vi "ReversedEngineering GetAdditionalTransitionStates.vi"(1 "SelStrings":string[](array[string]), 2 "StringConstant":string) -> (15 "AdditionalTransitionStates":string[](array[string]))   [LabVIEW 2020]
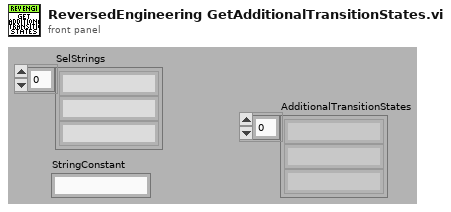
[diagram p1: front panel]
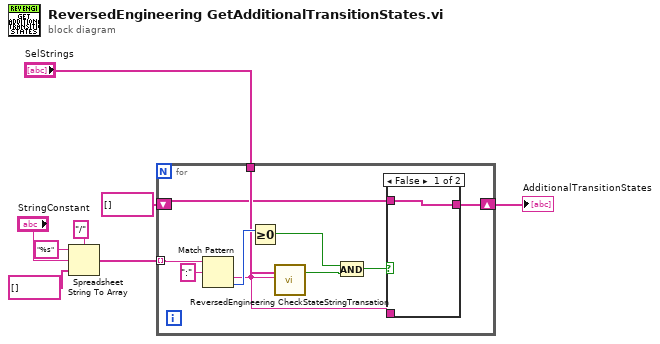
[diagram p0: block diagram]
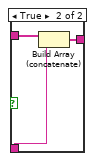
[diagram p2: hidden frame]
diagram:
  n1 = Spreadsheet String To Array(delimiter (Tab)="/", format string="%s", spreadsheet string="StringConstant", array type (2D Dbl)=string[] []) -> (array=w4:string[])
  n2 = for {
    tunnel: w4 -> [w17] mode=indexing
    tunnel: "SelStrings" -> [w15]
    shift-right: [w11] -> w1
    shift-left: string[] [] -> [w10]
    n3 = Match Pattern(string=w17, regular expression=":") -> (after substring=w9:string, offset past match=w16:i32)  [unwired: 3 out]
    n4 = Greater Or Equal To 0?(x=w16) -> (x >= 0?=w13:bool)
    n5 = call <resource>:"ReversedEngineering CheckStateStringTransation.vi"("SelStrings"=w15, "StringConstant"=w9) -> ("Found"=w14:bool)  [unwired: 2 in, 15 out]
    n6 = And(x=w13, y=w14) -> (x .and. y?=w12:bool)
    n7 = case shown="False" w12 {
      tunnel: [w19 w22] -> w11
      tunnel: w10 -> [w19 w21]
      tunnel: w9 -> [_ w20]
      frame False {
      }
      frame True {
        n8 = Build Array (concatenate)(w21, w20) -> (w22:string[])
      }
    }
  }
  "AdditionalTransitionStates" <- w1
